vi "Module Name--constant.vi"() -> (3 "Module Name":string)   [LabVIEW 2016, in "Impedance Data Acquisition and Decoding.lvlib"]
doc: "Return the name of the module that owns this VI. \n_____\nBased on Delacor QMH Project Template 5.0.0.82."
uses:
  Impedance Data Acquisition and Decoding.lvlib
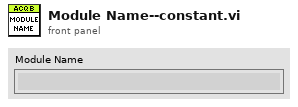
[diagram p1: front panel]
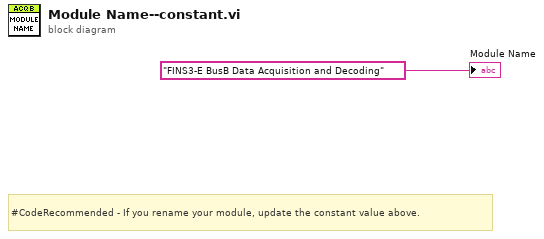
[diagram p0: block diagram]
diagram:
  # "#CodeRecommended - If you rename your module, update the constant value above."
  "Module Name" <- "FINS3-E BusB Data Acquisition and Decoding"
